vi "Parametri Controls.vi"() -> ()   [LabVIEW 2020]
panel:
  in  "Enum":enum16{""}(ring)
  in  "String Array":string[](array[string])
  in  "Control":T1(array[cluster])=[{"Device"=10, "Operation"=0, "Command/byte count"="OUTP:LOAD INF\nAPPL:SIN 1000,10,0"}, {"Device"=1, "Operation"=0, "Command/byte count"="HEAD OFF\nDAT:SOU CH1\nDAT:ENC ASCI\nDAT:WID 1\nDAT:STAR 1\nDAT:STOP 2500\nCURV?"}, {"Device"=1, "Operation"=1, "Command/byte count"="15000"}] {"Operation" items=["write", "read"]; "Device" items=["DSO"=1, "AWG"=10]}
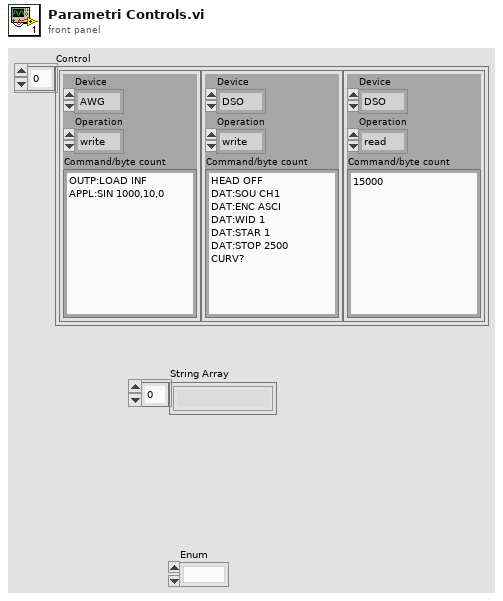
[diagram p1: front panel]
types:
  T1 = cluster{"Device":u16, "Operation":u16, "Command/byte count":string}[]
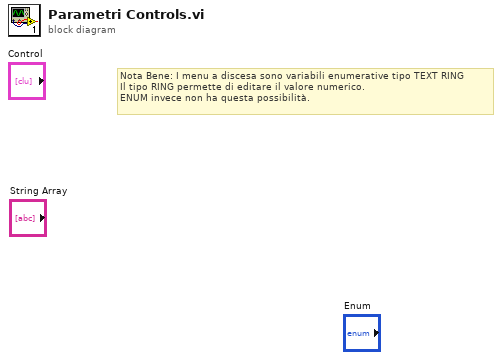
[diagram p0: block diagram]
diagram:
  # "Nota Bene: I menu a discesa sono variabili enumerative tipo TEXT RING\nIl tipo RING permette di editare il valore numerico.\nENUM invece non ha questa possibilità."
